vi "Or77200_AskPos.vi"(8 "error In":errorcluster caption="error out", 10 "Lambda":dbl caption="Longueur d'ondes (nm)" min=0.0 max=9999.0 step=0.1 format="%.1f") -> (0 "sortie d'erreur":errorcluster, 2 "Lambda Out":dbl min=0.0 max=9999.0 step=0.1 format="%.1f")   [LabVIEW 2019]
panel:
  in  "OK":bool
  # "Entrez la longueur d'ondes du monochromateur telle qu'indiquée sur le compteur\n\nAttention! : Le dernier chiffre est la position décimale (0,1 nm)"
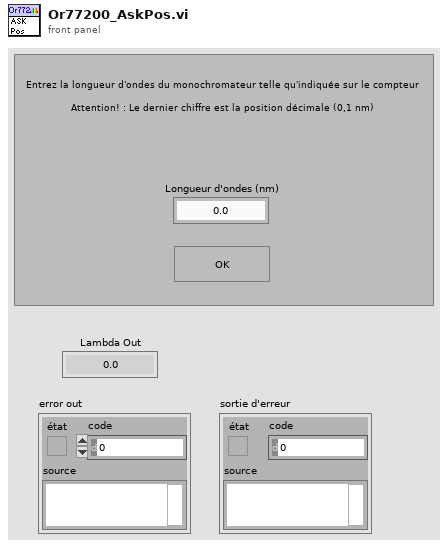
[diagram p1: front panel]
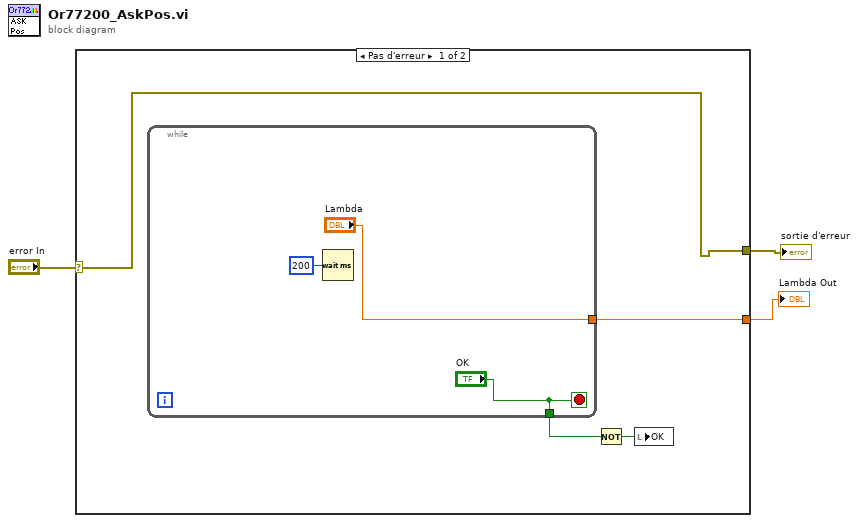
[diagram p0: block diagram]
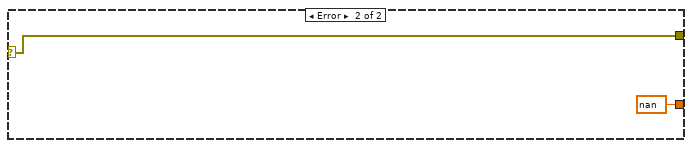
[diagram p2: hidden frame]
diagram:
  n1 = case shown="Pas d'erreur" "error In" {
    selector: "error In" -> [w4 w11]
    tunnel: [w5 nan ("Longueur d'ondes (nm)")] -> w3
    tunnel: [w4 w11] -> w1
    frame No Error {
      n2 = while {
        tunnel: ["OK"] -> w7
        tunnel: ["Lambda"] -> w5
        stop <- "OK" stop-if-true
        n3 = Wait (ms)(milliseconds to wait=u32 200 ("attente (ms)")) -> ()  [unwired: 1 out]
      }
      n4 = Not(x=w7) -> (.not. x?=w6:bool)
      n5 = local write "OK"(w6) -> ()
    }
    frame Error {
    }
  }
  "Lambda Out" <- w3
  "sortie d'erreur" <- w1
